vi "shutdown_DSC.vi"(0 "MoAgSy_Host":refnum<class "MoAgSy_Host.lvclass">, 5 "error in (no error)":errorcluster) -> (14 "dup_MoAgSy_Host":refnum<class "MoAgSy_Host.lvclass">, 19 "error out":errorcluster)   [LabVIEW 2009, in "MoAgSy.lvlib" / "MoAgSy_Host.lvclass"]
doc: "<B>public</B> Vi destroys DSC Monitor and DSC Var Manager\nof referenced Host.\n\nF.Berck@gsi.de\nGSI Darmstadt 2009"
uses:
  MoAgSy_Host.lvclass
  HGF_BaseClasses/HGF_Stop/HGF_Stop.lvclass
  MoAgSy_Host.lvclass/MoAgSy_Host.ctl
  HGF_BaseClasses/HGF_Event/HGF_Event.lvclass
  HGF_BaseClasses/HGF_TriggeredEvent/HGF_TriggeredEvent.lvclass
  HGF_BaseClasses/HGF_Factory/HGF_Factory.lvclass
  HGF_BaseClasses/HGF_ThreadPool/HGF_ThreadPool.lvclass
  HGF_BaseClasses/HGF_Reference/HGF_Reference.lvclass
panel:
  # "DSC"
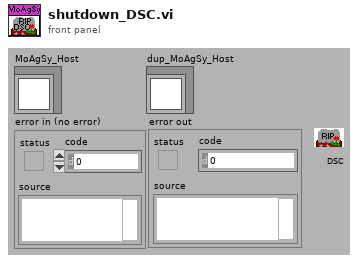
[diagram p1: front panel]
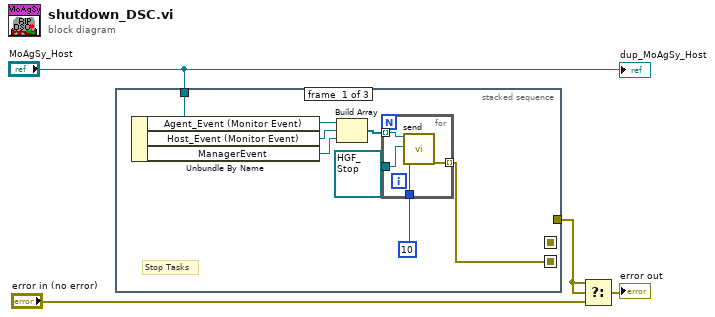
[diagram p0: block diagram]
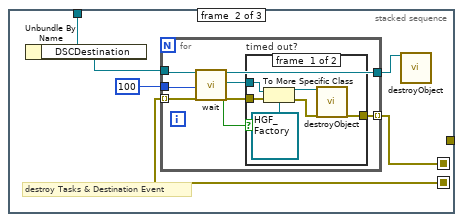
[diagram p2: hidden frame]
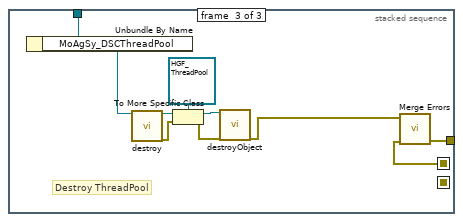
[diagram p4: hidden frame]
diagram:
  n1 = stacked-sequence {
    seq-local: [w5 _ _] -> [_ w18 _]
    seq-local: [_ w17 _] -> [_ _ w37]
    tunnel: "MoAgSy_Host" -> [w6 w19 w41]
    tunnel: [_ _ w38] -> w3
    frame #0 {
      # "Stop Tasks"
      n2 = Unbundle By Name(w6) -> ("Agent_Event (Monitor Event)"=w11:refnum<class "HGF_Event.lvclass">, "Host_Event (Monitor Event)"=w10:refnum<class "HGF_Event.lvclass">, "ManagerEvent"=w9:refnum<class "HGF_Event.lvclass">)
      n3 = Build Array(w11, w10, w9) -> (w8:refnum<class "HGF_Event.lvclass">[])
      n4 = for {
        tunnel: refnum<class "HGF_Stop.lvclass"> refnum ("HGF_BaseClasses.lvlib:HGF_Stop.lvclass") -> [w16]
        tunnel: w8 -> [w15] mode=indexing
        tunnel: 10 -> [w14]
        tunnel: [w13] -> w5 mode=indexing
        n5 = call-dynamic "send.vi"("HGF_Event"=w15, "Object"=w16, "timeout in ms (-1)"=w14) -> ("error out"=w13:errorcluster)  [unwired: 14 in, 2 out]
      }
    }
    frame #1 {
      # "destroy Tasks & Destination Event"
      n6 = Unbundle By Name(w19) -> ("DSCDestination"=w21:refnum<class "HGF_TriggeredEvent.lvclass">)
      n7 = for {
        tunnel: w21 -> [w30]
        tunnel: 100 ("msTimeout (-1)") -> [w29]
        tunnel: w18 -> [w28] mode=indexing
        tunnel: [w24] -> w22
        tunnel: [w23] -> w17 mode=indexing
        n8 = call-dynamic "wait.vi"("HGF_Event"=w30, "msTimeout (-1)"=w29, "error in (no error)"=w28) -> ("dup HGF_Event"=w24:refnum<class "HGF_TriggeredEvent.lvclass">, "Object"=w25:refnum<class>, "timed out"=w27:bool, "error out"=w26:errorcluster)  [unwired: 13 in]
        n9 = case "timed out?" shown="False" w27 {
          tunnel: w26 -> [w36 _]
          tunnel: w25 -> [w35 _]
          tunnel: [w31 _] -> w23
          frame #0 {
            n10 = To More Specific Class(target class=refnum<class "HGF_Factory.lvclass"> refnum ("HGF_BaseClasses.lvlib:HGF_Factory.lvclass"), reference=w35, error in=w36) -> (specific class reference=w33:refnum<class "HGF_Factory.lvclass">, error out=w32:errorcluster)
            n11 = call "destroyObject.vi"("HGF_Factory"=w33, "error in (no error)"=w32) -> ("error out"=w31:errorcluster)  [unwired: 17 in]
          }
          frame #1 {
          }
        }
      }
      n12 = call "destroyObject.vi"("HGF_Factory"=w22) -> ()  [unwired: 18 in, 1 out]
    }
    frame #2 {
      # "Destroy ThreadPool"
      n13 = Unbundle By Name(w41) -> ("MoAgSy_DSCThreadPool"=w40:refnum<class "HGF_Reference.lvclass">)
      n14 = call "destroy.vi"("HGF_Reference"=w40) -> ("Object"=w43:refnum<class>, "error out"=w46:errorcluster)  [unwired: 17 in]
      n15 = To More Specific Class(target class=refnum<class "HGF_ThreadPool.lvclass"> refnum ("HGF_BaseClasses.lvlib:HGF_ThreadPool.lvclass"), reference=w43, error in=w46) -> (specific class reference=w44:refnum<class "HGF_ThreadPool.lvclass">, error out=w42:errorcluster)
      n16 = call "destroyObject.vi"("HGF_Factory"=w44, "error in (no error)"=w42) -> ("error out"=w39:errorcluster)  [unwired: 17 out]
      n17 = call <vilib>:"Merge Errors.vi"("error array in"=w37, "error in 1 (no error)"=w39) -> ("error out"=w38:errorcluster)  [unwired: 5 in]
    }
  }
  n18 = Select(t=w3, s=w3, f="error in (no error)") -> (s? t:f=→"error out":errorcluster)
  "dup_MoAgSy_Host" <- "MoAgSy_Host"
